vi "GDevCon Omnibus.vi"() -> ()   [LabVIEW 2020, in "CTI-Scratchpad.lvlib"]
uses:
  CTI-Scratchpad.lvlib
  CTI/Error Reporting.ctl
  CTI/GPIO Number.ctl
  CTI/I2C Number.ctl
  CTI/ADC Number.ctl
  CTI-Peripheral/Character LCD/Position.ctl
  CTI/GPIO Direction.ctl
  CTI/Raw ADC.ctl
  CTI-Peripheral/Grove I2C LCD/Grove I2C LCD.lvclass
  CTI/Session/Session.lvclass
  CTI/VisaComms/VisaComms.lvclass
  CTI/CTI.lvlib
  CTI-Peripheral/Character LCD/Char LCD.lvclass
panel:
  in  "Home":bool
  in  "Clear":bool
  in  "LED":bool
  in  "PWM Enable":bool
  out "Act. Freq":sgl format="%.4f"
  out "Act. Duty":sgl format="%_6f"
  in  "Frequency":sgl(slide) scale=10.0..500000.0
  in  "Duty":sgl(slide) scale=0.0..1.0
  out "Mic":dbl(knob) scale=0.0..4095.0
  out "PIR":bool
  out "Button":bool
  in  "Position":T1
  in  "Goto":bool
  out "Potentiometer":dbl(knob) scale=0.0..1.0
  in  "Write LCD":bool
  in  "LCD Text":string
  in  "Stop":bool
  in  "I2C Baud":u32=400000 format="%.0p"
  in  "Mic AI":T2=1
  in  "Pot AI":T2
  in  "SDA GPIO":T3=6
  in  "SCL GPIO":T3=7
  in  "I2C #":T4=1
  in  "PIR GPIO":T3=28
  in  "Buzzer GPIO":T3=18
  in  "LED GPIO":T3=20
  in  "Button GPIO":T3=16
  in  "Error Checking":T5
  in  "VISA resource name":refnum<visa-resource-name>="COM5"
  # "Buzzer"
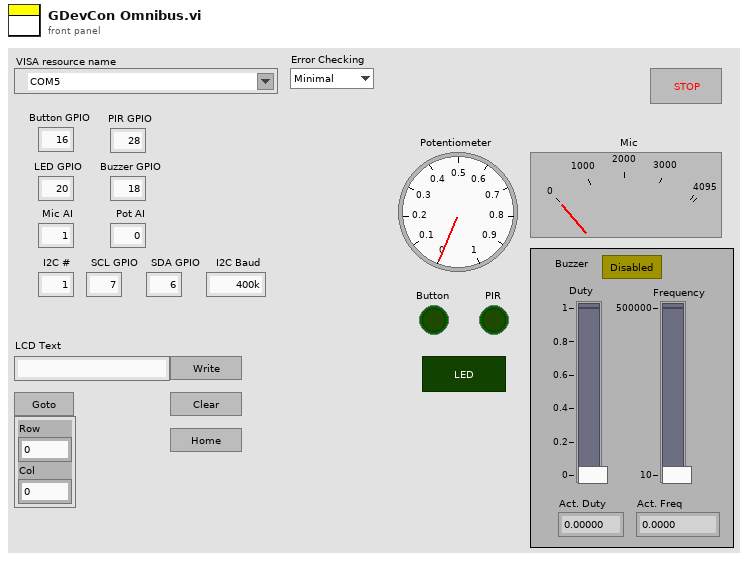
[diagram p1: front panel]
types:
  T1 = typedef "CTI-Peripheral.lvlib/Char LCD.lvclass/Position.ctl" = cluster{"Row":u8, "Col":u8}
  T2 = typedef "CTI.lvlib/ADC Number.ctl" = i8
  T3 = typedef "CTI.lvlib/GPIO Number.ctl" = i8
  T4 = typedef "CTI.lvlib/I2C Number.ctl" = i8
  T5 = typedef "CTI.lvlib/Error Reporting.ctl" = enum16{"Minimal", "Moderate", "Full"}
  T6 = typedef "CTI.lvlib/GPIO Direction.ctl" = enum16{"In", "Out"}
  T7 = typedef "CTI.lvlib/Raw ADC.ctl" = u16
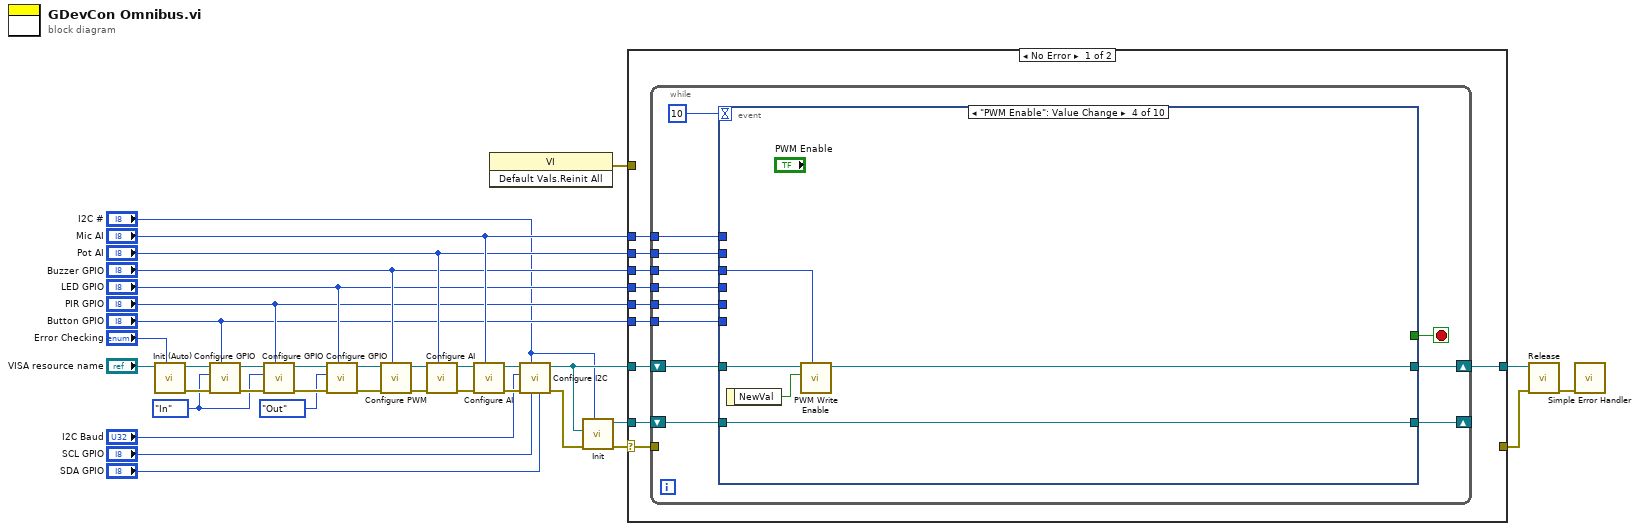
[diagram p0: block diagram]
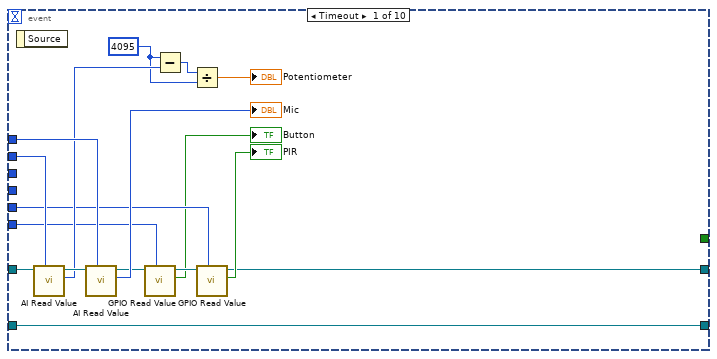
[diagram p2: hidden frame]
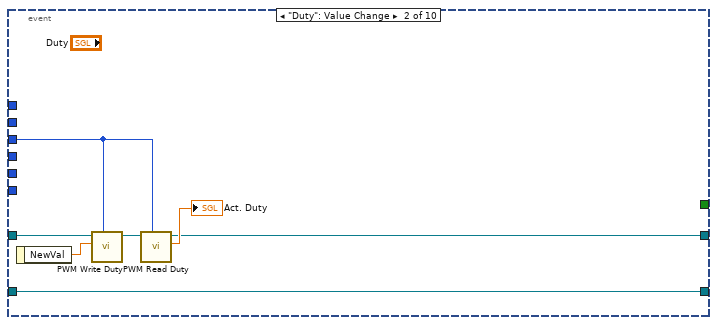
[diagram p3: hidden frame]
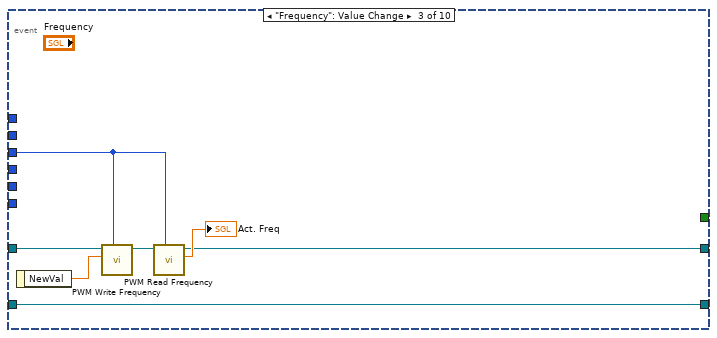
[diagram p4: hidden frame]
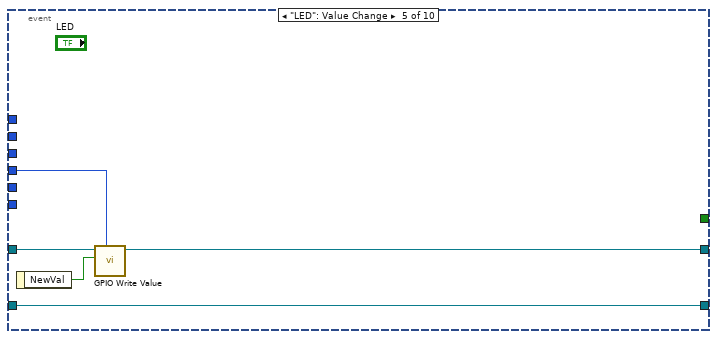
[diagram p5: hidden frame]
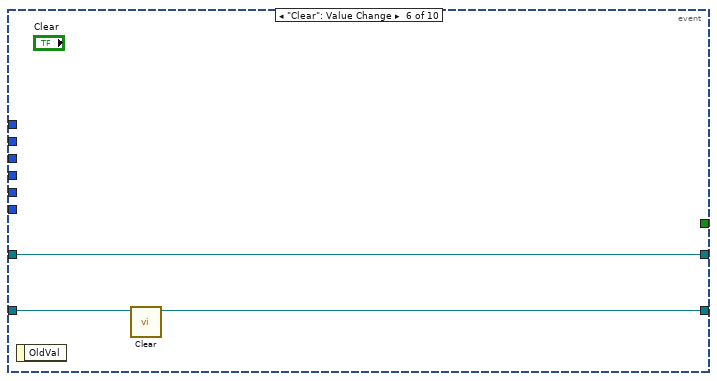
[diagram p6: hidden frame]
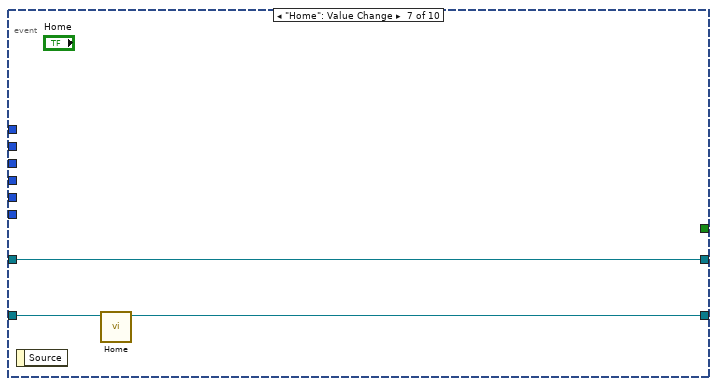
[diagram p7: hidden frame]
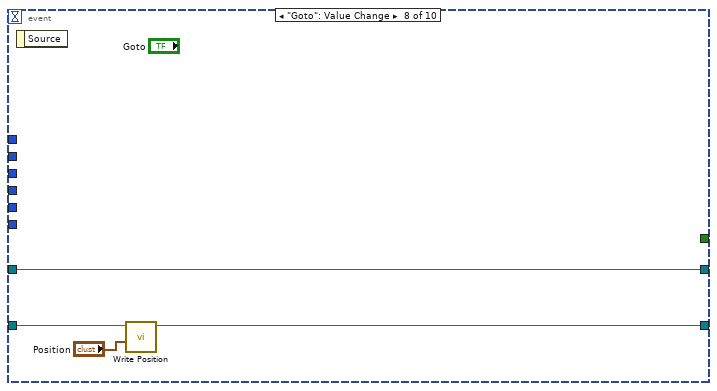
[diagram p8: hidden frame]
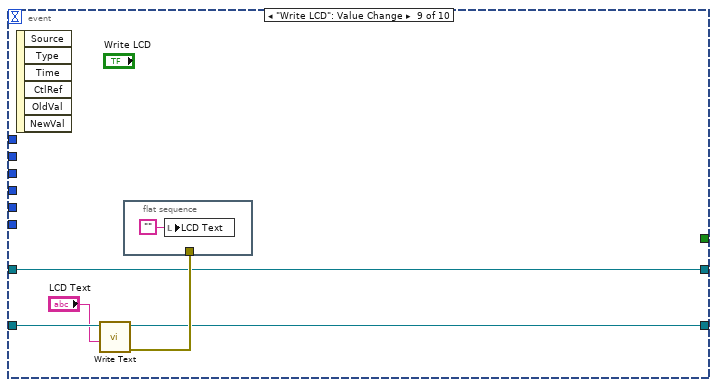
[diagram p9: hidden frame]
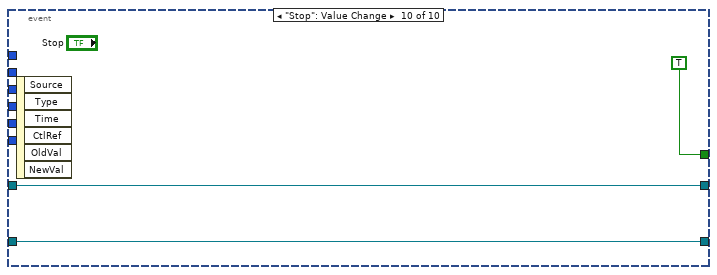
[diagram p10: hidden frame]
diagram:
  w26 = GPIO_Direction."In" ("GPIO Direction")
  n1 = call "Init (Auto).vi"("Error Checking (Full)"="Error Checking", "VISA resource name"="VISA resource name") -> ("error out"=w33:errorcluster, "Session"=w32:refnum<class "Session.lvclass">)  [unwired: 7 in, 1 out]
  n2 = call "Configure GPIO.vi"("GPIO #"="Button GPIO", "error in (no error)"=w33, "GPIO Direction"=w26, "Session in"=w32) -> ("error out"=w28:errorcluster, "Session out"=w27:refnum<class "Session.lvclass">)  [unwired: 6 in]
  n3 = call "Configure GPIO.vi"("GPIO #"="PIR GPIO", "error in (no error)"=w28, "GPIO Direction"=w26, "Session in"=w27) -> ("error out"=w36:errorcluster, "Session out"=w25:refnum<class "Session.lvclass">)  [unwired: 6 in]
  n4 = call "Configure GPIO.vi"("GPIO #"="LED GPIO", "error in (no error)"=w36, "GPIO Direction"=GPIO_Direction."Out", "Session in"=w25) -> ("error out"=w30:errorcluster, "Session out"=w31:refnum<class "Session.lvclass">)  [unwired: 6 in]
  n5 = call "Configure PWM.vi"("GPIO #"="Buzzer GPIO", "error in (no error)"=w30, "Session in"=w31) -> ("error out"=w21:errorcluster, "Session out"=w20:refnum<class "Session.lvclass">)  [unwired: 7 in]
  n6 = call "Configure AI.vi"("ADC #"="Pot AI", "error in (no error)"=w21, "Session in"=w20) -> ("error out"=w19:errorcluster, "Session out"=w18:refnum<class "Session.lvclass">)  [unwired: 7 in]
  n7 = call "Configure AI.vi"("ADC #"="Mic AI", "error in (no error)"=w19, "Session in"=w18) -> ("error out"=w16:errorcluster, "Session out"=w17:refnum<class "Session.lvclass">)  [unwired: 7 in]
  n8 = invoke class="VI" method="Default Vals.Reinit All"() -> (error out=w2:errorcluster)  [unwired: 3 in, 2 out]
  n9 = call "Configure I2C.vi"("SDA GPIO"="SDA GPIO", "SCL GPIO"="SCL GPIO", "I2C #"="I2C #", "error in (no error)"=w16, "Baud"="I2C Baud", "Session in"=w17) -> ("error out"=w24:errorcluster, "Session out"=w12:refnum<class "Session.lvclass">)  [unwired: 4 in]
  n10 = call "Init.vi"("I2C #"="I2C #", "error in (no error)"=w24, "Session In"=w12) -> ("error out"=w13:errorcluster, "Grove I2C LCD out"=w14:refnum<class "Grove I2C LCD.lvclass">)  [unwired: 7 in]
  n11 = case shown="No Error" w13 {
    selector: w13 -> [w45 w119]
    tunnel: w14 -> [w46 _]
    tunnel: w12 -> [w44 w120]
    tunnel: [w43 w120] -> w11
    tunnel: [_ w119] -> w10
    tunnel: "Mic AI" -> [w42 _]
    tunnel: "Pot AI" -> [w41 _]
    tunnel: "Buzzer GPIO" -> [w40 _]
    tunnel: "LED GPIO" -> [w39 _]
    tunnel: "PIR GPIO" -> [w38 _]
    tunnel: "Button GPIO" -> [w37 _]
    tunnel: w2 -> [_ _]
    frame No Error {
      n12 = while {
        tunnel: w45 -> [_]
        shift-right: [w56] -> w43
        shift-left: w44 -> [w57]
        shift-right: [w55] -> _
        shift-left: w46 -> [w54]
        tunnel: w42 -> [w52]
        tunnel: w41 -> [w51]
        tunnel: w40 -> [w50]
        tunnel: w39 -> [w49]
        tunnel: w38 -> [w48]
        tunnel: w37 -> [w47]
        stop <- w53 stop-if-true
        n13 = event shown="[3] \"PWM Enable\": Value Change" {
          selector: _ -> [_ _ _ _ _ _ _ _ _ _]
          dyn-events: _ -> [_ _ _ _ _ _ _ _ _ _]
          timeout: 10 -> [_ _ _ _ _ _ _ _ _ _]
          tunnel: w57 -> [w74 w81 w88 w93 w98 w102 w105 w109 w113 w118]
          tunnel: [w59 w77 w85 w90 w95 w102 w105 w109 w113 w118] -> w56
          tunnel: [w75 w82 w89 w94 w99 w101 w103 w106 w112 w117] -> w55
          tunnel: w54 -> [w75 w82 w89 w94 w99 w100 w104 w107 w111 w117]
          tunnel: [_ _ _ _ _ _ _ _ _ TRUE] -> w53
          tunnel: w52 -> [w71 _ _ _ _ _ _ _ _ _]
          tunnel: w51 -> [w73 _ _ _ _ _ _ _ _ _]
          tunnel: w50 -> [_ w76 w84 w91 _ _ _ _ _ _]
          tunnel: w49 -> [_ _ _ _ w96 _ _ _ _ _]
          tunnel: w48 -> [w62 _ _ _ _ _ _ _ _ _]
          tunnel: w47 -> [w64 _ _ _ _ _ _ _ _ _]
          event Timeout {
            w67 = T7 4095 ("y")
            n14 = event-data() -> ()  [unwired: 1 in, 1 out]
            n15 = call "AI Read Value.vi"("ADC #"=w73, "Session in"=w74) -> ("Value"=w69:T7, "Session out"=w72:refnum<class "Session.lvclass">)  [unwired: 7 in, 1 out]
            n16 = call "AI Read Value.vi"("ADC #"=w71, "Session in"=w72) -> ("Value"=→"Mic":T7, "Session out"=w65:refnum<class "Session.lvclass">)  [unwired: 7 in, 1 out]
            n17 = call "GPIO Read Value.vi"("GPIO #"=w64, "Session in"=w65) -> ("Value"=→"Button":bool, "Session out"=w63:refnum<class "Session.lvclass">)  [unwired: 7 in, 1 out]
            n18 = Subtract(x=w67, y=w69) -> (x-y=w68:T7)
            n19 = Divide(x=w68, y=w67) -> (x/y=→"Potentiometer":dbl)
            n20 = call "GPIO Read Value.vi"("GPIO #"=w62, "Session in"=w63) -> ("Value"=→"PIR":bool, "Session out"=w59:refnum<class "Session.lvclass">)  [unwired: 7 in, 1 out]
          }
          event "Duty": Value Change {
            n21 = event-data() -> ("NewVal"=w80:sgl)  [unwired: 1 in]
            n22 = call "PWM Write Duty.vi"("GPIO #"=w76, "Duty % (0-1)"=w80, "Session in"=w81) -> ("Session out"=w79:refnum<class "Session.lvclass">)  [unwired: 7 in, 1 out]
            n23 = call "PWM Read Duty.vi"("GPIO #"=w76, "Session in"=w79) -> ("Duty % (0-1)"=→"Act. Duty":sgl, "Session out"=w77:refnum<class "Session.lvclass">)  [unwired: 7 in, 1 out]
          }
          event "Frequency": Value Change {
            n24 = event-data() -> ("NewVal"=w83:sgl)  [unwired: 1 in]
            n25 = call "PWM Write Frequency.vi"("GPIO #"=w84, "Frequency Hz"=w83, "Session in"=w88) -> ("Session out"=w87:refnum<class "Session.lvclass">)  [unwired: 7 in, 1 out]
            n26 = call "PWM Read Frequency.vi"("GPIO #"=w84, "Session in"=w87) -> ("Frequency Hz"=→"Act. Freq":sgl, "Session out"=w85:refnum<class "Session.lvclass">)  [unwired: 7 in, 1 out]
          }
          event "PWM Enable": Value Change {
            n27 = event-data() -> ("NewVal"=w92:bool)  [unwired: 1 in]
            n28 = call "PWM Write Enable.vi"("GPIO #"=w91, "Enable"=w92, "Session in"=w93) -> ("Session out"=w90:refnum<class "Session.lvclass">)  [unwired: 7 in, 1 out]
          }
          event "LED": Value Change {
            n29 = event-data() -> ("NewVal"=w97:bool)  [unwired: 1 in]
            n30 = call "GPIO Write Value.vi"("GPIO #"=w96, "Value"=w97, "Session in"=w98) -> ("Session out"=w95:refnum<class "Session.lvclass">)  [unwired: 7 in, 1 out]
          }
          event "Clear": Value Change {
            n31 = event-data() -> ()  [unwired: 1 in, 1 out]
            n32 = call-dynamic "Clear.vi"("Character LCD in"=w100) -> ("Character LCD out"=w101:refnum<class "Grove I2C LCD.lvclass">)  [unwired: 9 in, 1 out]
          }
          event "Home": Value Change {
            n33 = event-data() -> ()  [unwired: 1 in, 1 out]
            n34 = call-dynamic "Home.vi"("Character LCD in"=w104) -> ("Character LCD out"=w103:refnum<class "Grove I2C LCD.lvclass">)  [unwired: 9 in, 1 out]
          }
          event "Goto": Value Change {
            n35 = event-data() -> ()  [unwired: 1 in, 1 out]
            n36 = call-dynamic "Write Position.vi"("Position"="Position", "Grove I2C LCD I in"=w107) -> ("Grove I2C LCD I out"=w106:refnum<class "Grove I2C LCD.lvclass">)  [unwired: 8 in, 1 out]
          }
          event "Write LCD": Value Change {
            n37 = event-data() -> ()  [unwired: 1 in, 6 out]
            n38 = call-dynamic "Write Text.vi"("Text"="LCD Text", "Character LCD in"=w111) -> ("error out"=w114:errorcluster, "Character LCD out"=w112:refnum<class "Grove I2C LCD.lvclass">)  [unwired: 8 in]
            n39 = flat-sequence {
              tunnel: w114 -> [_]
              frame #0 {
                n40 = local write "LCD Text"("" ("LCD Text")) -> ()
              }
            }
          }
          event "Stop": Value Change {
            n41 = event-data() -> ()  [unwired: 1 in, 6 out]
          }
        }
      }
    }
    frame Error {
    }
  }
  n42 = call-dynamic "Release.vi"("error in (no error)"=w10, "Session in"=w11) -> ("error out"=w9:errorcluster)  [unwired: 9 in]
  n43 = call <vilib>:"Simple Error Handler.vi"("error in (no error)"=w9) -> ()  [unwired: 4 in, 5 out]
